vi "Parse Phone Number.vi"(11 "Phone# In":string) -> (3 "Phone# Out":string)   [LabVIEW 2013]
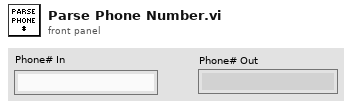
[diagram p1: front panel]
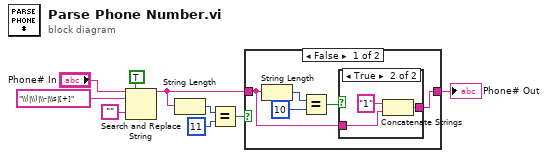
[diagram p0: block diagram]
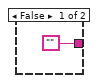
[diagram p2: hidden frame]
diagram:
  n1 = Search and Replace String(replace all?=TRUE ("replace all? (F)"), input string="Phone# In", search string="\\(|\\)|\\-|\\s|[+]" ("regular expression"), replace string="") -> (result string=w4:string)  [unwired: 4 in, 3 out]
  n2 = String Length(string=w4) -> (length=w3:i32)
  n3 = Equal?(x=w3, y=11) -> (x = y?=w5:bool)
  n4 = case shown="False" w5 {
    tunnel: w4 -> [w11 w19]
    tunnel: [w10 w19] -> w1
    frame False {
      n5 = String Length(string=w11) -> (length=w14:i32)
      n6 = Equal?(x=w14, y=10) -> (x = y?=w12:bool)
      n7 = case shown="True" w12 {
        tunnel: w11 -> [_ w18]
        tunnel: ["" w16] -> w10
        frame False {
        }
        frame True {
          n8 = Concatenate Strings("1" ("string"), w18) -> (w16:string)
        }
      }
    }
    frame True {
    }
  }
  "Phone# Out" <- w1
